vi "Timer_Get.vi"(8 "Pass_Through_Time":dbl=-1.0 format="%33.4f", 11 "TIMER":T1 {"Accumulated TIme" format="%13.5p"; "StartTime" format="%13.5p"}) -> (3 "CurrentTImer":dbl)   [LabVIEW 2019, in "Trajectory_Library.lvlib"]
doc: "Get the current time from the timer. If the clock is running it is derived from the current system clock the start time stored in the timer class. If the clock is not running, then return the time when it was last stopped.\n\nInputs:\n - Timer -- The Timer data cluster\n\nOutputs:\n - CurrentTimer -- Current time value for this timer in seconds"
uses:
  Trajectory_Library.lvlib
  TypeDef/TIMER.ctl
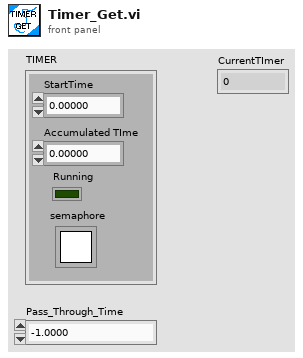
[diagram p1: front panel]
types:
  T1 = typedef "Trajectory_Library.lvlib/TIMER.ctl" = cluster{"StartTime":dbl, "Accumulated TIme":dbl, "Running":bool, "semaphore":T2}
  T2 = typedef "Semaphore RefNum" = refnum<k1>
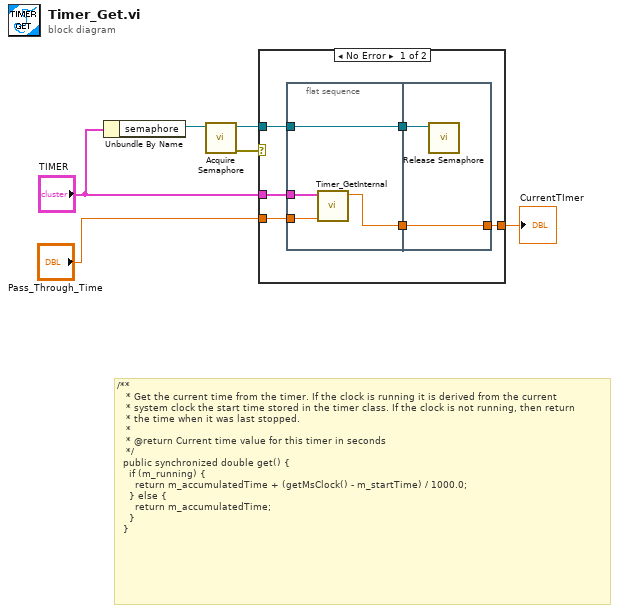
[diagram p0: block diagram]
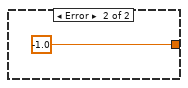
[diagram p2: hidden frame]
diagram:
  # "/**\n   * Get the current time from the timer. If the clock is running it is derived from the current\n   * system clock the start time stored in the timer class. If the clock is not running, then return\n   * the time when it was last stopped.\n   *\n   * @return Current time value for this timer in seconds\n   */\n  public synchronized double get() {\n    if (m_running) {\n      return m_accumulatedTime + (getMsClock() - m_startTime) / 1000.0;\n    } else {\n      return m_accumulatedTime;\n    }\n  }"
  n1 = Unbundle By Name("TIMER") -> ("semaphore"=w4:T2)
  n2 = call <vilib>:"Acquire Semaphore.vi"("semaphore"=w4) -> ("error out"=w3:errorcluster, "semaphore out"=w2:T2)  [unwired: 4 in, 1 out]
  n3 = case shown="No Error" w3 {
    tunnel: [w11 -1.0 ("Accumulated TIme")] -> w6
    tunnel: "TIMER" -> [w12 _]
    tunnel: w2 -> [w8 _]
    tunnel: "Pass_Through_Time" -> [w7 _]
    frame No Error {
      n4 = flat-sequence {
        tunnel: w12 -> [w16]
        tunnel: [w15] -> w10
        tunnel: [w14] -> w9
        tunnel: w8 -> [w14]
        tunnel: w7 -> [w13]
        tunnel: [w18] -> w11
        tunnel: w10 -> [w18]
        tunnel: w9 -> [w17]
        frame #0 {
          n5 = call "Timer_GetInternal.vi"("Pass_Through_Time"=w13, "TIMER"=w16) -> ("CurrentTImer"=w15:dbl)  [unwired: 8 in, 1 out]
        }
        frame #1 {
          n6 = call <vilib>:"Release Semaphore.vi"("semaphore"=w17) -> ()  [unwired: 5 in, 2 out]
        }
      }
    }
    frame Error {
    }
  }
  "CurrentTImer" <- w6
